vi "Eval.vi"(8 "error in (no error)":errorcluster, 11 "muExpr in":refnum<class "muExpr.lvclass">) -> (0 "error out":errorcluster, 2 "Result":dbl format="%#_13g", 3 "muExpr out":refnum<class "muExpr.lvclass">)   [LabVIEW 2015, in "muParser.lvlib" / "muExpr.lvclass"]
uses:
  muExpr.lvclass
  muExpr.lvclass/muExpr.ctl
  mupLib/mupCheckError.vi
  muParser.lvlib
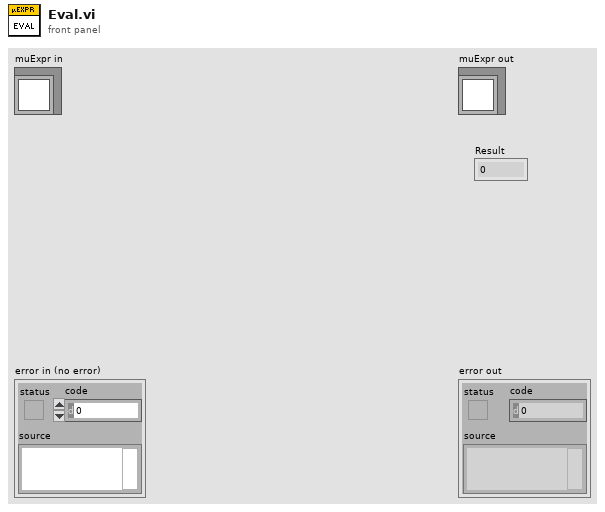
[diagram p1: front panel]
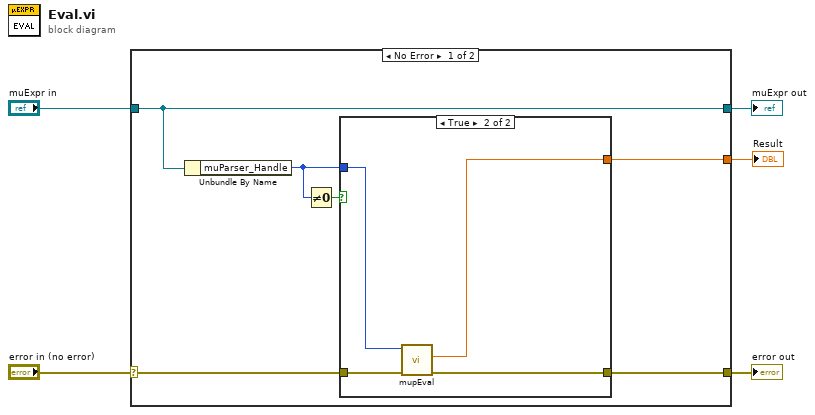
[diagram p0: block diagram]
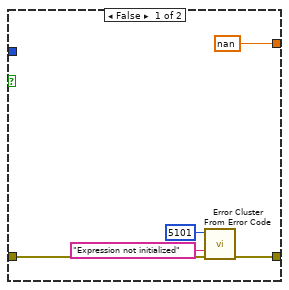
[diagram p2: hidden frame]
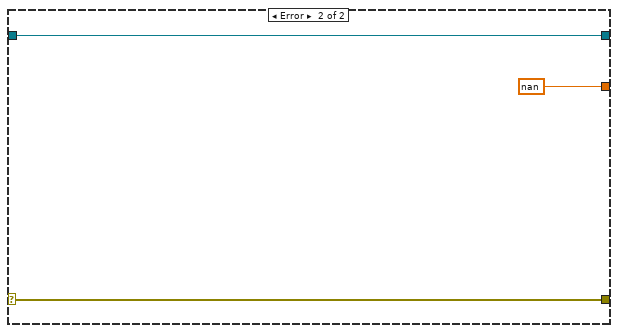
[diagram p3: hidden frame]
diagram:
  n1 = case shown="No Error" "error in (no error)" {
    selector: "error in (no error)" -> [w10 w23]
    tunnel: [w7 w23] -> w4
    tunnel: [w11 w22] -> w2
    tunnel: "muExpr in" -> [w11 w22]
    tunnel: [w6 nan ("return type")] -> w1
    frame No Error {
      n2 = Unbundle By Name(w11) -> ("muParser_Handle"=w9:u64)
      n3 = Not Equal To 0?(x=w9) -> (x != 0?=w8:bool)
      n4 = case shown="True" w8 {
        tunnel: w10 -> [w15 w19]
        tunnel: [w14 w17] -> w7
        tunnel: [nan ("return type") w18] -> w6
        tunnel: w9 -> [_ w20]
        frame False {
          n5 = call <vilib>:"Error Cluster From Error Code.vi"("error in (no error)"=w15, "error message (\"\")"="Expression not initialized" ("error message (\"\")"), "error code (0)"=5101) -> ("error out"=w14:errorcluster)  [unwired: 6 in]
        }
        frame True {
          n6 = call "mupEval.vi"("error in (no error)"=w19, "hParser in"=w20) -> ("error out"=w17:errorcluster, "result"=w18:dbl)  [unwired: 7 in, 1 out]
        }
      }
    }
    frame Error {
    }
  }
  "error out" <- w4
  "muExpr out" <- w2
  "Result" <- w1
